vi "Generate Events.vi"(10 "Flags":bool[](array[boolean])) -> (3 "Events":T1={"Touch"=FALSE, "Ball out"=FALSE, "id touch"=0.0, "Ball out of \nVision"=FALSE, "Ball inside \nGoalie area"=FALSE, "Robot not responding"=FALSE, "Robots responding status"=[1.0, 1.0, 1.0, 1.0, 1.0, 1.0], "Enemy Ball \nPossession"=FALSE, "Pass State"=FALSE, "id end of pass"=0.0, "Kick"=FALSE, "Id ini Possession"=0.0, "Ball Possesion"=FALSE, "Id Possesion"=0.0})   [LabVIEW 2017]
uses:
  Util/Events/Events.ctl
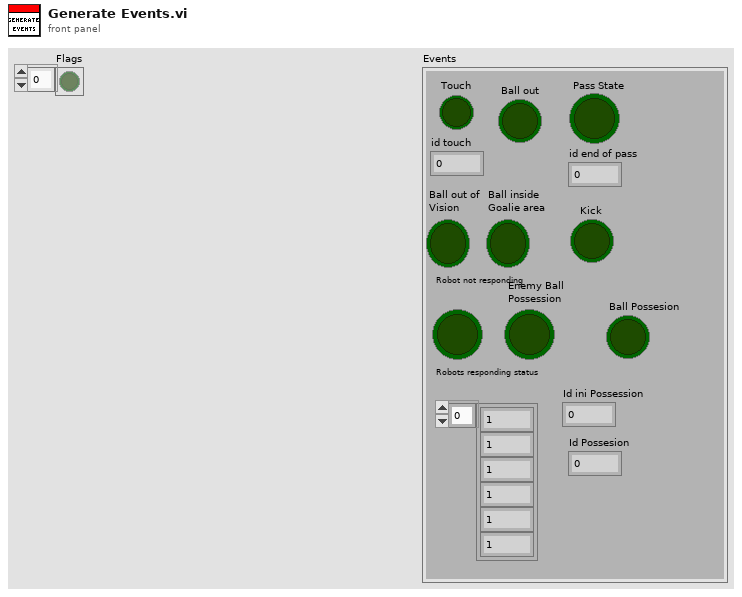
[diagram p1: front panel]
types:
  T1 = typedef "Events.ctl" = cluster{"Touch":bool, "Ball out":bool, "id touch":dbl, "Ball out of \nVision":bool, "Ball inside \nGoalie area":bool, "Robot not responding":bool, "Robots responding status":dbl[], "Enemy Ball \nPossession":bool, "Pass State":bool, "id end of pass":dbl, "Kick":bool, "Id ini Possession":dbl, "Ball Possesion":bool, "Id Possesion":dbl}
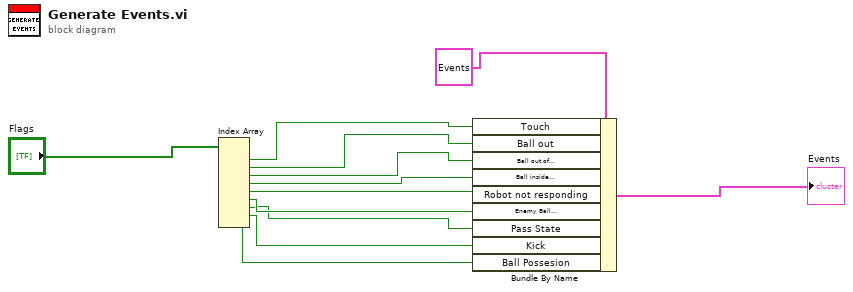
[diagram p0: block diagram]
diagram:
  n1 = Index Array(array="Flags") -> (element #1=w11:bool, element #2=w10:bool, element #3=w9:bool, element #4=w8:bool, element #5=w7:bool, element #6=w6:bool, element #7=w5:bool, element #8=w4:bool, element #9=w1:bool)  [unwired: 9 in]
  n2 = Bundle By Name(cluster=T1 {"Touch"=FALSE, "Ball out"=FALSE, "id touch"=0.0, "Ball out of \nVision"=FALSE, "Ball inside \nGoalie area"=FALSE, "Robot not responding"=FALSE, "Robots responding status"=[1.0, 1.0, 1.0, 1.0, 1.0, 1.0], "Enemy Ball \nPossession"=FALSE, "Pass State"=FALSE, "id end of pass"=0.0, "Kick"=FALSE, "Id ini Possession"=0.0, "Ball Possesion"=FALSE, "Id Possesion"=0.0} ("Events"), "Touch"=w11, "Ball out"=w10, "Ball out of \nVision"=w9, "Ball inside \nGoalie area"=w8, "Robot not responding"=w7, "Enemy Ball \nPossession"=w6, "Pass State"=w5, "Kick"=w4, "Ball Possesion"=w1) -> (→"Events":T1)
